vi "prepareDialogMethod.vi"(8 "error in (no error)":errorcluster, 10 "dialogVIRefnum":refnum<vi>, 11 "ViewThisComponent in":refnum<class "ViewThisComponent.lvclass">) -> (0 "error out":errorcluster, 3 "ViewThisComponent out":refnum<class "ViewThisComponent.lvclass">)   [LabVIEW 2016, in "ViewThisComponent.lvclass"]
doc: "Sets the value of the \"view\" control on each of the views in the subpanel to a View object equipped with the valid viewUserEvent."
uses:
  ViewThisComponent.lvclass
  C:/ApeironSW/CMP_UserEvents/ComponentTemplateCore/ComponentModel/ComponentModel/View/View.lvclass
  ComponentTemplateCore/ComponentModel/ComponentModel/View/View.lvclass/View.ctl
  ViewThisComponent.lvclass/ViewThisComponent.ctl
  ComponentTemplateCore/ComponentModel/ComponentModel/View/View.lvclass
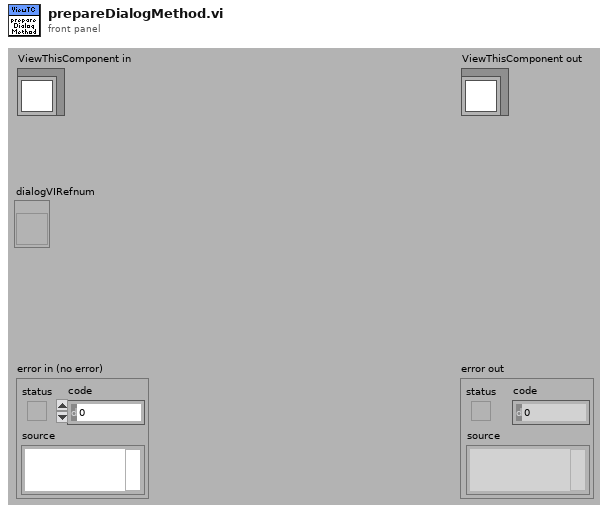
[diagram p1: front panel]
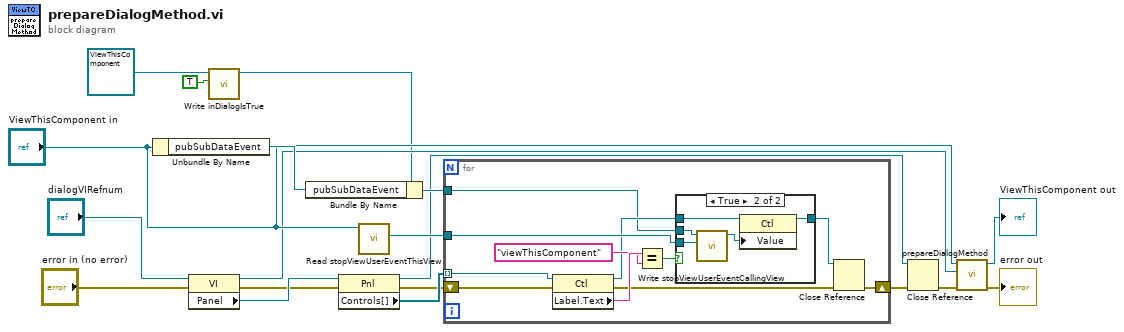
[diagram p0: block diagram]
diagram:
  n1 = Unbundle By Name("ViewThisComponent in") -> ("pubSubDataEvent"=w16:refnum<class "PubSubDataEvent.lvclass">)
  n2 = property class="VI"(reference="dialogVIRefnum", error in="error in (no error)") -> (reference out=w4:refnum<vi>, error out=w8:errorcluster, "Panel"=w11:refnum<vi>)
  n3 = call "Write inDialogIsTrue.vi"("indialogIsTrue"=TRUE, "View in"=refnum<class "ViewThisComponent.lvclass"> refnum ("ViewThisComponent.lvclass")) -> ("View out"=w2:refnum<class "ViewThisComponent.lvclass">)  [unwired: 9 in]
  n4 = Bundle By Name(cluster=w2, "pubSubDataEvent"=w16) -> (w17:refnum<class "ViewThisComponent.lvclass">)
  n5 = property class="Pnl"(reference=w11, error in=w8) -> (reference out=w9:refnum<vi>, error out=w7:errorcluster, "Controls[]"=w10:refnum<vi>[])
  n6 = call "Read stopViewUserEventThisView.vi"("View in"="ViewThisComponent in") -> ("stopViewUserEventThisView"=w18:refnum<user-event>)  [unwired: 9 in, 1 out]
  n7 = for {
    tunnel: w10 -> [w30] mode=indexing
    tunnel: w18 -> [w26]
    shift-right: [w21] -> w6
    shift-left: w7 -> [w23]
    tunnel: w17 -> [w20]
    n8 = property class="Ctl"(reference=w30, error in=w23) -> (reference out=w24:refnum<vi>, error out=w22:errorcluster, "Label.Text"=w29:string)
    n9 = Equal?(x=w29, y="viewThisComponent") -> (x = y?=w27:bool)
    n10 = case shown="True" w27 {
      tunnel: w26 -> [_ w34]
      tunnel: [w31 w35] -> w25
      tunnel: w24 -> [w31 w36]
      tunnel: w20 -> [_ w33]
      frame False {
      }
      frame True {
        n11 = call "Write stopViewUserEventCallingView.vi"("stopViewUserEventCallingView"=w34, "View in"=w33) -> ("View out"=w32:refnum<class "ViewThisComponent.lvclass">)  [unwired: 9 in]
        n12 = property class="Ctl"(reference=w36, "Value"=w32) -> (reference out=w35:refnum<vi>)  [unwired: 1 in, 1 out]
      }
    }
    n13 = Close Reference(reference=w25, error in (no error)=w22) -> (error out=w21:errorcluster)
  }
  n14 = Close Reference(reference=w9, error in (no error)=w6) -> (error out=w14:errorcluster)
  n15 = call-parent "prepareDialogMethod.vi"("error in (no error)"=w14, "dialogVIRefnum"=w4, "View in"="ViewThisComponent in") -> ("error out"=→"error out":errorcluster, "View out"=→"ViewThisComponent out":refnum<class "ViewThisComponent.lvclass">)  [unwired: 7 in]
